vi "LAC Cmd114_Cam trig_mode.vi"(6 "R/W (F:Read)":bool, 7 "timeout(ms)":u32=500, 8 "error in":errorcluster, 10 "Trig_mode":enum16{"OFF", "ON"}(ring), 11 "VISA name in":refnum<visa-resource-name>) -> (0 "error out":errorcluster, 1 "readout":string, 3 "VISA name out":refnum<visa-resource-name>)   [LabVIEW 2014]
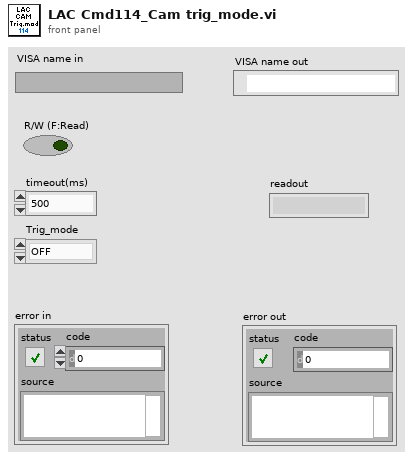
[diagram p1: front panel]
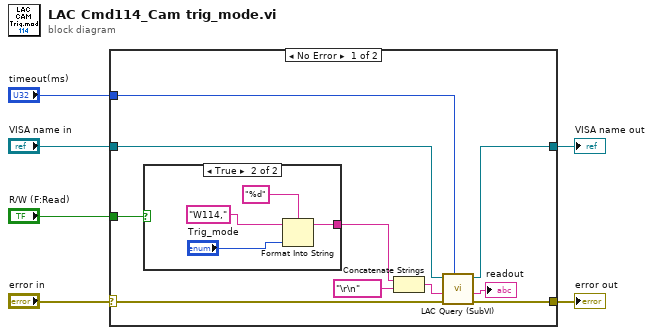
[diagram p0: block diagram]
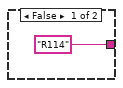
[diagram p2: hidden frame]
diagram:
  n1 = case shown="No Error" "error in" {
    selector: "error in" -> [w12 w23]
    tunnel: "VISA name in" -> [w14 w22]
    tunnel: [w16 w22] -> w5
    tunnel: [w15 w23] -> w4
    tunnel: "timeout(ms)" -> [w13 _]
    tunnel: "R/W (F:Read)" -> [w7 _]
    frame No Error {
      n2 = case shown="True" w7 {
        tunnel: ["R114" ("string") w18] -> w8
        frame False {
        }
        frame True {
          n3 = Format Into String(format string="%d", initial string="W114," ("string"), "Trig_mode") -> (resulting string=w18:string)  [unwired: 1 in, 1 out]
        }
      }
      n4 = Concatenate Strings(w8, "\r\n" ("write buffer")) -> (w10:string)
      n5 = call "LAC Query (SubVI).vi"("timeout(ms)"=w13, "error in"=w12, "Command"=w10, "VISA name in"=w14) -> ("error out"=w15:errorcluster, "read buffer"=→"readout":string, "VISA name out"=w16:refnum<visa-resource-name>)  [unwired: 5 in]
    }
    frame Error {
    }
  }
  "VISA name out" <- w5
  "error out" <- w4
